vi "Set Power Supplies On.vi"(8 "error in (no error)":errorcluster, 11 "Driver Test in":refnum<class "Driver Test.lvclass">) -> (0 "error out":errorcluster)   [LabVIEW 2015, in "Instrument Setup.lvclass"]
uses:
  Instrument Setup.lvclass
  Driver Test/Driver Test.lvclass
  Test Class/Test Class.lvclass
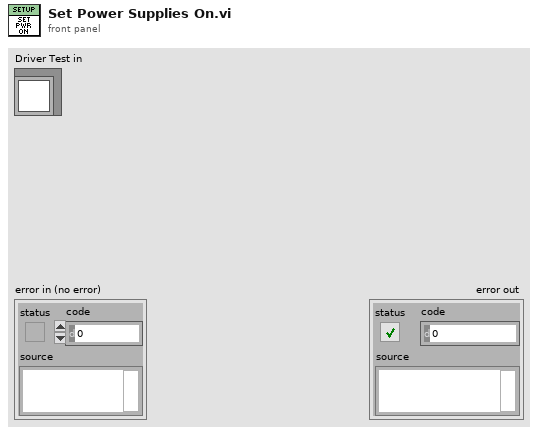
[diagram p1: front panel]
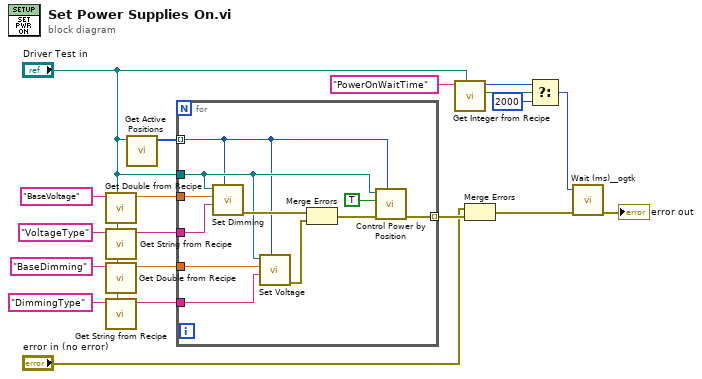
[diagram p0: block diagram]
diagram:
  n1 = call "Get Double from Recipe.vi"("Test Class in"="Driver Test in", "Name"="BaseVoltage") -> ("Value"=w14:dbl)  [unwired: 7 in, 2 out]
  n2 = call "Get String from Recipe.vi"("Test Class in"="Driver Test in", "Name"="VoltageType") -> ("Value"=w12:string)  [unwired: 7 in, 2 out]
  n3 = call "Get Double from Recipe.vi"("Test Class in"="Driver Test in", "Name"="BaseDimming") -> ("Value"=w13:dbl)  [unwired: 7 in, 2 out]
  n4 = call "Get String from Recipe.vi"("Test Class in"="Driver Test in", "Name"="DimmingType") -> ("Value"=w11:string)  [unwired: 7 in, 2 out]
  n5 = call "Get Active Positions.vi"("Test Class in"="Driver Test in") -> ("Active Positions"=w10:u32[])  [unwired: 9 in, 1 out]
  n6 = for {
    tunnel: "Driver Test in" -> [w23]
    tunnel: w14 -> [w28]
    tunnel: w13 -> [w26]
    tunnel: w12 -> [w27]
    tunnel: w11 -> [w25]
    tunnel: w10 -> [w22] mode=indexing
    tunnel: [w20] -> w9 mode=indexing
    n7 = call "Set Dimming.vi"("Position"=w22, "Dimming Type"=w27, "Dim Level"=w28, "Driver Test in"=w23) -> ("error out"=w30:errorcluster)  [unwired: 7 in]
    n8 = call "Set Voltage.vi"("Position"=w22, "Voltage Type"=w25, "Voltage"=w26, "Driver Test in"=w23) -> ("error out"=w29:errorcluster)  [unwired: 7 in]
    n9 = Merge Errors(w30, w29) -> (w24:errorcluster)
    n10 = call "Control Power by Position.vi"("Position"=w22, "error in (no error)"=w24, "Power On?"=TRUE, "Driver Test in"=w23) -> ("error out"=w20:errorcluster)  [unwired: 7 in]
  }
  n11 = call "Get Integer from Recipe.vi"("Test Class in"="Driver Test in", "Name"="PowerOnWaitTime") -> ("found?"=w4:bool, "Value"=w3:i32)  [unwired: 7 in, 1 out]
  n12 = Merge Errors("error in (no error)", w9) -> (w8:errorcluster)
  n13 = Select(t=w3, s=w4, f=2000) -> (s? t:f=w1:i32)
  n14 = call <userlib>:"Wait (ms)__ogtk.vi"("error in (no error)"=w8, "milliseconds to wait"=w1) -> ("error out"=→"error out":errorcluster)  [unwired: 8 in, 1 out]
